vi "Translator SD Card Library File Class.vi"(0 "Input":variant=variant("Function Name"=variant(string "Strip Path"), "Input Datatypes"=variant(string[] ["error", "int"]), "Inputs"=variant(string[] ["error in", "x"]), "Node refnum"=variant(refnum<vi> refnum), "Output Datatypes"=variant(string[] ["int"]), "Outputs"=variant(string[] ["a"])), 11 "error in (no error)":errorcluster) -> (4 "Output":variant=variant("Defines"=variant(string[] []), "Includes"=variant(string[] []), "Replaced Code"=variant(string "/* LabVIEW system function 'Strip Path' not found. */")), 15 "error out":errorcluster)   [LabVIEW 2014, in "LabVIEW Universal Transcriptor SD Card Library.lvlib" / "File.lvclass"]
doc: "Translator for SD card. This library is inteded just for one SD card, not multiple, because arduino functios are written over global object, there is no need to have class implementation."
uses:
  File.lvclass
panel:
  out "Outputs":string[](array[string])
  out "Inputs":string[](array[string])
  out "Output Datatypes":string[](array[string])
  out "Input Datatypes":string[](array[string])
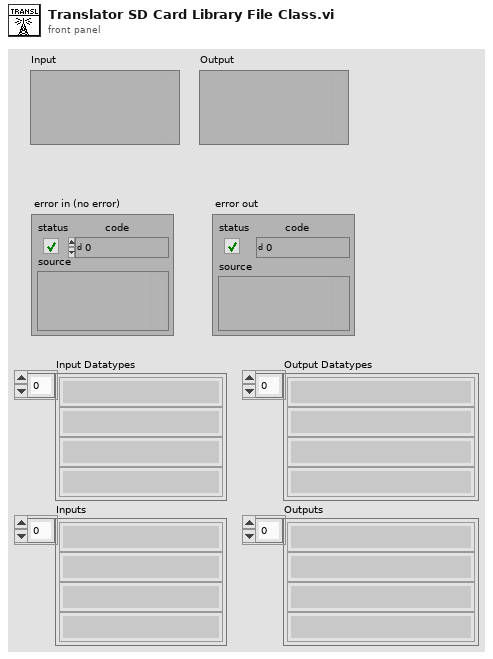
[diagram p1: front panel]
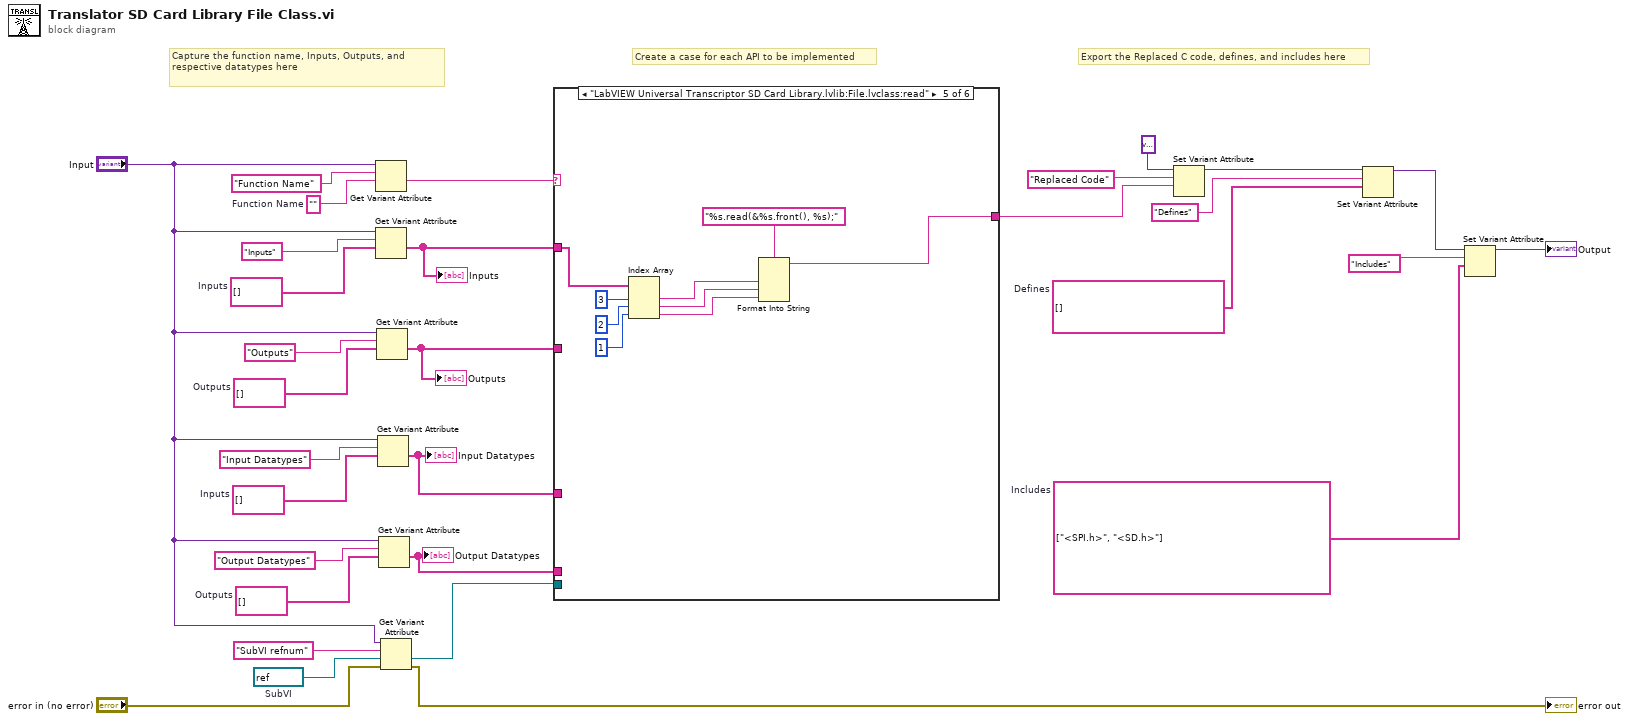
[diagram p0: block diagram]
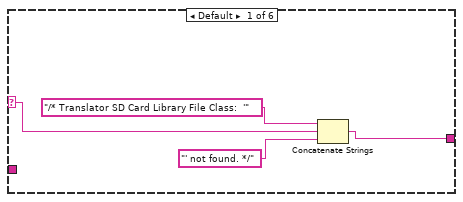
[diagram p2: hidden frame]
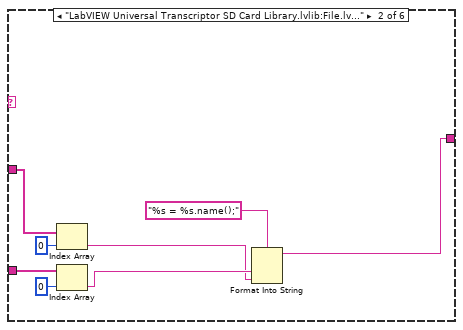
[diagram p3: hidden frame]
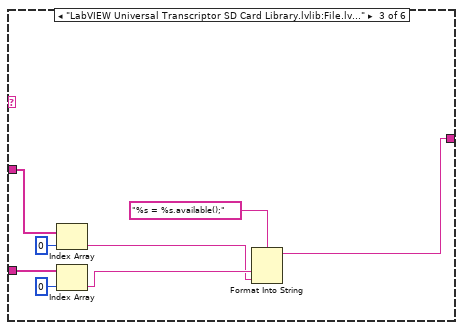
[diagram p4: hidden frame]
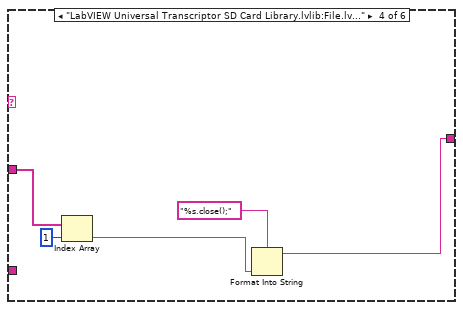
[diagram p5: hidden frame]
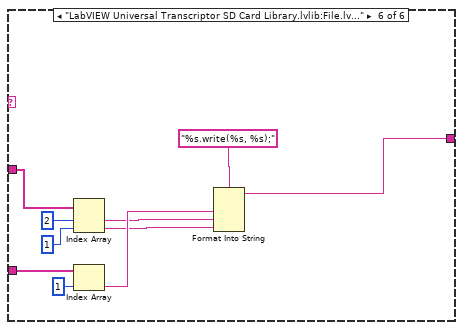
[diagram p6: hidden frame]
diagram:
  w7 = refnum<vi> refnum  # SubVI
  w4 = string[] []  # Defines
  w17 = string[] []  # Outputs
  w18 = string[] []  # Inputs
  w3 = string[] ["<SPI.h>", "<SD.h>"]  # Includes
  w27 = string[] []  # Outputs
  w28 = string[] []  # Inputs
  w29 = ""  # Function Name
  # "Capture the function name, Inputs, Outputs, and respective datatypes here"
  # "Export the Replaced C code, defines, and includes here"
  # "Create a case for each API to be implemented"
  n1 = Get Variant Attribute(Variant="Input", name="Function Name", default value (empty Variant)=w29) -> (value=w24:string)  [unwired: 1 in, 3 out]
  n2 = Get Variant Attribute(Variant="Input", name="Inputs", default value (empty Variant)=w28) -> (value=w14:string[])  [unwired: 1 in, 3 out]
  "Inputs" <- w14
  n3 = Get Variant Attribute(Variant="Input", name="Outputs", default value (empty Variant)=w27) -> (value=w15:string[])  [unwired: 1 in, 3 out]
  "Outputs" <- w15
  n4 = Get Variant Attribute(Variant="Input", name="Input Datatypes", default value (empty Variant)=w18) -> (value=w10:string[])  [unwired: 1 in, 3 out]
  "Input Datatypes" <- w10
  n5 = Get Variant Attribute(Variant="Input", name="Output Datatypes", default value (empty Variant)=w17) -> (value=w5:string[])  [unwired: 1 in, 3 out]
  "Output Datatypes" <- w5
  n6 = Get Variant Attribute(Variant="Input", name="SubVI refnum", default value (empty Variant)=w7, error in="error in (no error)") -> (value=w6:refnum<vi>, error out=→"error out":errorcluster)  [unwired: 2 out]
  n7 = case shown="\"LabVIEW Universal Transcriptor SD Card Library.lvlib:File.lvclass:read\"" w24 {
    selector: w24 -> [w34 _ _ _ _ _]
    tunnel: [w32 w37 w45 w53 w63 w70] -> w23
    tunnel: w14 -> [_ w36 w44 w52 w62 w66]
    tunnel: w15 -> [_ w42 w50 _ _ w74]
    tunnel: w10 -> [_ _ _ _ _ _]
    tunnel: w6 -> [_ _ _ _ _ _]
    tunnel: w5 -> [_ _ _ _ _ _]
    frame Default {
      n8 = Concatenate Strings("/* Translator SD Card Library File Class:  '", w34, "' not found. */") -> (w32:string)
    }
    frame "LabVIEW Universal Transcriptor SD Card Library.lvlib:File.lvclass:name" {
      n9 = Index Array(array=w36, index=0) -> (element=w38:string)
      n10 = Index Array(array=w42, index=0) -> (element=w39:string)
      n11 = Format Into String(format string="%s = %s.name();" ("name"), w39, w38) -> (resulting string=w37:string)  [unwired: 2 in, 1 out]
    }
    frame "LabVIEW Universal Transcriptor SD Card Library.lvlib:File.lvclass:available" {
      n12 = Index Array(array=w44, index=0) -> (element=w46:string)
      n13 = Index Array(array=w50, index=0) -> (element=w47:string)
      n14 = Format Into String(format string="%s = %s.available();" ("name"), w47, w46) -> (resulting string=w45:string)  [unwired: 2 in, 1 out]
    }
    frame "LabVIEW Universal Transcriptor SD Card Library.lvlib:File.lvclass:close" {
      n15 = Index Array(array=w52, index=1) -> (element=w54:string)
      n16 = Format Into String(format string="%s.close();" ("name"), w54) -> (resulting string=w53:string)  [unwired: 2 in, 1 out]
    }
    frame "LabVIEW Universal Transcriptor SD Card Library.lvlib:File.lvclass:read" {
      n17 = Index Array(array=w62, index #1=3 ("index"), index #2=2 ("index"), index #3=1 ("index")) -> (element #1=w57:string, element #2=w60:string, element #3=w59:string)
      n18 = Format Into String(format string="%s.read(&%s.front(), %s);", w57, w60, w59) -> (resulting string=w63:string)  [unwired: 2 in, 1 out]
    }
    frame "LabVIEW Universal Transcriptor SD Card Library.lvlib:File.lvclass:write" {
      n19 = Index Array(array=w66, index #1=2 ("index"), index #2=1 ("index")) -> (element #1=w71:string, element #2=w67:string)
      n20 = Index Array(array=w74, index=1) -> (element=w73:string)
      n21 = Format Into String(format string="%s.write(%s, %s);", w73, w71, w67) -> (resulting string=w70:string)  [unwired: 2 in, 1 out]
    }
  }
  n22 = Set Variant Attribute(Variant=variant ("variant"), name="Replaced Code", value=w23) -> (Variant out=w13:variant)  [unwired: 1 in, 2 out]
  n23 = Set Variant Attribute(Variant=w13, name="Defines", value=w4) -> (Variant out=w12:variant)  [unwired: 1 in, 2 out]
  n24 = Set Variant Attribute(Variant=w12, name="Includes", value=w3) -> (Variant out=→"Output":variant)  [unwired: 1 in, 2 out]
